vi "G2CPU graph.vi"(8 "error in (no error)":errorcluster, 9 "C":refnum<class "2D Array f32.lvclass">, 10 "B":refnum<class "2D Array f32.lvclass">, 11 "A":refnum<class "2D Array f32.lvclass">) -> (0 "error out":errorcluster, 3 "real out":dbl)   [LabVIEW 2020]
uses:
  <vilib>/Natan Biesmans/G2CPU GPU and CPU HPC Toolkit/G2CPU Libraries/Arrays/2DArray/f32/2D Array f32.lvclass
  C:/Program Files/National Instruments/LabVIEW 2020/vi.lib/Natan Biesmans/G2CPU GPU and CPU HPC Toolkit/G2CPU Libraries/Arrays/Array/Array Prototype.lvclass
  <vilib>/Natan Biesmans/G2CPU GPU and CPU HPC Toolkit/ArrayFire Driver/TypeDefs/MatMulFunctions.ctl
  f39f69ef-cdc5-4b54-9a41-a91f8f42218f.vi
  292a3864-d678-49fd-9f52-7b3d0f58df6a.vi
  250d4844-f155-4ba4-9ba6-bda3ee80715b.vi
  d9e87bb7-38f7-4789-9499-842ecc6160f5.vi
  f39f69ef-cdc5-4b54-9a41-a91f8f42218f.vi/741da8b7-e115-4068-b6c8-09c0e3e4c17b.vi
  f39f69ef-cdc5-4b54-9a41-a91f8f42218f.vi/6ccb08d3-06fa-4eaa-a429-be2dd0e65cf6.vi
  f39f69ef-cdc5-4b54-9a41-a91f8f42218f.vi/40092443-1088-494b-9937-e6fe53927ce9.vi
  292a3864-d678-49fd-9f52-7b3d0f58df6a.vi/4890056b-ab47-4030-8abd-bbdacd5197a6.vi
  G2CPU_ADD_Float.vi/20c5033d-e34b-4680-b71c-a1cccc2834c5.vi
  G2CPU_ADD_Float.vi/86f0bec7-6e21-4a72-bbfd-824d9a80339c.vi
  250d4844-f155-4ba4-9ba6-bda3ee80715b.vi/8b1efca8-af3b-4021-8086-ccf117d769be.vi
  d9e87bb7-38f7-4789-9499-842ecc6160f5.vi/de34b5ac-b6d0-48d4-a9e3-cf41f219f91c.vi
  G2CPU_ADD_Float.vi/20c5033d-e34b-4680-b71c-a1cccc2834c5.vi/c3df215f-16d2-4e03-9745-9dd0f506ba18.vi
  G2CPU_ADD_Float.vi/20c5033d-e34b-4680-b71c-a1cccc2834c5.vi/c20e9e56-711a-4e3b-9a46-427845f2f903.vi
  G2CPU_ADD_Float.vi/20c5033d-e34b-4680-b71c-a1cccc2834c5.vi/80faa85e-9fb6-4da7-8f9b-44b1f9974ab2.vi
  G2CPU_ADD_Float.vi/20c5033d-e34b-4680-b71c-a1cccc2834c5.vi/730f6c57-5c0b-4ee9-b61e-75067b25222b.vi
  G2CPU_ADD_Float.vi/86f0bec7-6e21-4a72-bbfd-824d9a80339c.vi/2c12aba4-aacf-4d7a-adbe-039f6155a93e.vi
  G2CPU_ADD_Float.vi/86f0bec7-6e21-4a72-bbfd-824d9a80339c.vi/f38cccb2-46f6-49f0-a8d6-9da0c88ff6f3.vi
  G2CPU_ADD_Float.vi/86f0bec7-6e21-4a72-bbfd-824d9a80339c.vi/ac1e884d-1009-4464-9d84-e30609b15cc4.vi
  G2CPU_ADD_Float.vi/86f0bec7-6e21-4a72-bbfd-824d9a80339c.vi/b0150bb8-c0d1-462d-a788-37cf62685507.vi
  G2CPU_ADD_Float.vi/86f0bec7-6e21-4a72-bbfd-824d9a80339c.vi/12ac66bb-3c71-4165-9bea-8297abbfa9f1.vi
  G2CPU_ADD_Float.vi/20c5033d-e34b-4680-b71c-a1cccc2834c5.vi/c3df215f-16d2-4e03-9745-9dd0f506ba18.vi/601f24f8-2999-4f98-8030-64fd8876c127.vi
  G2CPU_ADD_Float.vi/20c5033d-e34b-4680-b71c-a1cccc2834c5.vi/c3df215f-16d2-4e03-9745-9dd0f506ba18.vi/e9745307-5113-4780-954c-71ccc9de0add.vi
  G2CPU_ADD_Float.vi/20c5033d-e34b-4680-b71c-a1cccc2834c5.vi/c20e9e56-711a-4e3b-9a46-427845f2f903.vi/c4afee3a-d58b-473f-ba2d-ee94fd2b49f4.vi
  G2CPU_ADD_Float.vi/20c5033d-e34b-4680-b71c-a1cccc2834c5.vi/80faa85e-9fb6-4da7-8f9b-44b1f9974ab2.vi/601f24f8-2999-4f98-8030-64fd8876c127.vi
  G2CPU_ADD_Float.vi/20c5033d-e34b-4680-b71c-a1cccc2834c5.vi/80faa85e-9fb6-4da7-8f9b-44b1f9974ab2.vi/e9745307-5113-4780-954c-71ccc9de0add.vi
  G2CPU_ADD_Float.vi/86f0bec7-6e21-4a72-bbfd-824d9a80339c.vi/ac1e884d-1009-4464-9d84-e30609b15cc4.vi/601f24f8-2999-4f98-8030-64fd8876c127.vi
  G2CPU_ADD_Float.vi/86f0bec7-6e21-4a72-bbfd-824d9a80339c.vi/ac1e884d-1009-4464-9d84-e30609b15cc4.vi/e9745307-5113-4780-954c-71ccc9de0add.vi
  G2CPU_ADD_Float.vi/86f0bec7-6e21-4a72-bbfd-824d9a80339c.vi/b0150bb8-c0d1-462d-a788-37cf62685507.vi/c5d3260c-dece-4fee-b11d-39452a92268b.vi
  G2CPU_ADD_Float.vi/86f0bec7-6e21-4a72-bbfd-824d9a80339c.vi/b0150bb8-c0d1-462d-a788-37cf62685507.vi/c5d3260c-dece-4fee-b11d-39452a92268b.vi/1a23f98f-393f-4176-8983-7f1ab824c539.vi
  <vilib>/Natan Biesmans/G2CPU GPU and CPU HPC Toolkit/G2CPU Libraries/Arrays/1DArray/f32/1D Array f32.lvclass
  <vilib>/Natan Biesmans/G2CPU GPU and CPU HPC Toolkit/G2CPU Libraries/Arrays/SubVI/Lock Arrays.vi
  <vilib>/Natan Biesmans/G2CPU GPU and CPU HPC Toolkit/G2CPU Libraries/Arrays/Array/G2CPU Get Array Pointer.vi
  <vilib>/Natan Biesmans/G2CPU GPU and CPU HPC Toolkit/ArrayFire Driver/VIs/gemm.vi
  <vilib>/Natan Biesmans/G2CPU GPU and CPU HPC Toolkit/G2CPU Libraries/Arrays/Array/G2CPU Unlock Array.vi
  <vilib>/Natan Biesmans/G2CPU GPU and CPU HPC Toolkit/G2CPU Libraries/Arrays/Array/G2CPU Release Array.vi
  <vilib>/Natan Biesmans/G2CPU GPU and CPU HPC Toolkit/G2CPU Libraries/Arrays/Array/G2CPU Set Array Pointer.vi
  <vilib>/Natan Biesmans/G2CPU GPU and CPU HPC Toolkit/G2CPU Libraries/Arrays/Array/G2CPU Lock Array.vi
  <vilib>/Natan Biesmans/G2CPU GPU and CPU HPC Toolkit/ArrayFire Driver/VIs/abs.vi
  <vilib>/Natan Biesmans/G2CPU GPU and CPU HPC Toolkit/ArrayFire Driver/VIs/Run as Multi Device.vi
  <vilib>/Natan Biesmans/G2CPU GPU and CPU HPC Toolkit/G2CPU Libraries/Manage Environment/Find AF DLL.vi
  <vilib>/Natan Biesmans/G2CPU GPU and CPU HPC Toolkit/ArrayFire Driver/subvi/Error Converter (ErrCode or Status).vi
  <vilib>/Natan Biesmans/G2CPU GPU and CPU HPC Toolkit/ArrayFire Driver/VIs/cast.vi
  <vilib>/Natan Biesmans/G2CPU GPU and CPU HPC Toolkit/G2CPU Libraries/Arrays/SubVI/is 2D.vi
  <vilib>/Natan Biesmans/G2CPU GPU and CPU HPC Toolkit/ArrayFire Driver/VIs/add.vi
  <vilib>/Natan Biesmans/G2CPU GPU and CPU HPC Toolkit/ArrayFire Driver/VIs/log.vi
  <vilib>/Natan Biesmans/G2CPU GPU and CPU HPC Toolkit/ArrayFire Driver/VIs/max all.vi
  <vilib>/Natan Biesmans/G2CPU GPU and CPU HPC Toolkit/G2CPU Libraries/Arrays/Array/Array Prototype.lvclass
  <vilib>/Natan Biesmans/G2CPU GPU and CPU HPC Toolkit/G2CPU Libraries/Arrays/DataTypes/f32/f32.lvclass
  <vilib>/Natan Biesmans/G2CPU GPU and CPU HPC Toolkit/G2CPU Libraries/Arrays/2DArray/2D Array Prototype.lvclass
  <vilib>/Natan Biesmans/G2CPU GPU and CPU HPC Toolkit/ArrayFire Driver/AF.lvlib
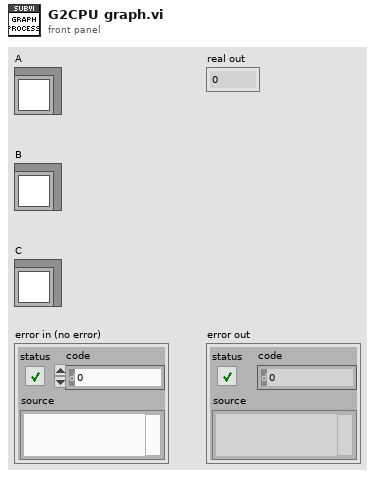
[diagram p1: front panel]
types:
  T1 = typedef "AF.lvlib/MatMulFunctions.ctl" = u32
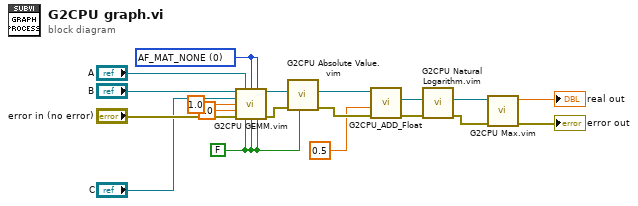
[diagram p0: block diagram]
diagram:
  w10 = T1 0 items=["AF_MAT_NONE"=0, "AF_MAT_TRANS"=1, "AF_MAT_CTRANS"=2, "AF_MAT_CONJ"=4, "AF_MAT_UPPER"=32, "AF_MAT_LOWER"=64, "AF_MAT_DIAG_UNIT"=128, "AF_MAT_SYM"=512, "AF_MAT_POSDEF"=1024, "AF_MAT_ORTHOG"=2048, "AF_MAT_TRI_DIAG"=4096, "AF_MAT_BLOCK_DIAG"=8192] ("optRhs")
  w3 = FALSE ("Auto Release Array A (Enabled)")
  n1 = call "G2CPU GEMM.vim"("Array B"="B", "Array A"="A", "opA"=w10, "opB"=w10, "Array C"="C", "alpha"=sgl 1.0, "beta"=sgl 0.0, "error in (no error)"="error in (no error)", "Auto Release Array A (Enabled)"=w3, "Auto Release Array B (Enabled)"=w3, "Auto Release Array C (Enabled)"=w3) -> ("Array Out"=w12:refnum<class "2D Array f32.lvclass">, "error out"=w15:errorcluster)  [unwired: 3 in]
  n2 = call "G2CPU Absolute Value.vim"("Auto Release (Enabled)"=w3, "error in (no error)"=w15, "Array in"=w12) -> ("error out"=w11:errorcluster, "Array Result"=w2:refnum<class "2D Array f32.lvclass">)  [unwired: 7 in]
  n3 = call "G2CPU_ADD_Float.vi"("error in (no error)"=w11, "Array rhs"=sgl 0.5, "Array lhs"=w2) -> ("error out"=w16:errorcluster, "Array Result"=w13:refnum<class "2D Array f32.lvclass">)  [unwired: 7 in]
  n4 = call "G2CPU Natural Logarithm.vim"("error in (no error)"=w16, "Array in"=w13) -> ("error out"=w17:errorcluster, "Array Result"=w4:refnum<class "2D Array f32.lvclass">)  [unwired: 8 in]
  n5 = call "G2CPU Max.vim"("error in (no error)"=w17, "Array First"=w4) -> ("error out"=→"error out":errorcluster, "real out"=→"real out":dbl)  [unwired: 7 in, 1 out]
